vi "triggerModbus.vi"(8 "error in (no error)":errorcluster, 11 "Model in":refnum<class "Model.lvclass">) -> (0 "error out":errorcluster, 3 "Model out":refnum<class "Model.lvclass">)   [LabVIEW 2016, in "Model.lvclass"]
uses:
  Model.lvclass
  Model.lvclass/Model.ctl
  Resources/FPGA/FPGA.lvclass
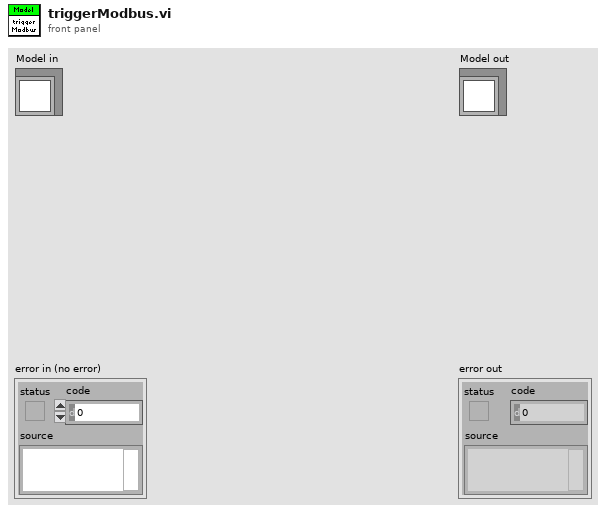
[diagram p1: front panel]
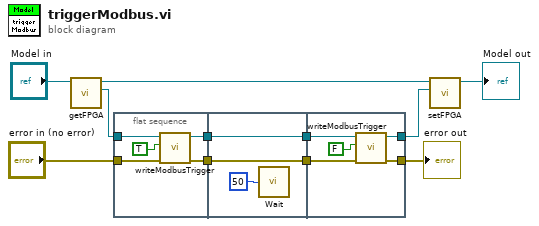
[diagram p0: block diagram]
diagram:
  n1 = call "getFPGA.vi"("Model in"="Model in") -> ("FPGA"=w8:refnum<class "FPGA.lvclass">, "Model out"=w10:refnum<class "Model.lvclass">)  [unwired: 9 in]
  n2 = flat-sequence {
    tunnel: w8 -> [w16]
    tunnel: [w15] -> w6
    tunnel: "error in (no error)" -> [w13]
    tunnel: [w12] -> w2
    tunnel: [w18] -> w7
    tunnel: w6 -> [w18]
    tunnel: [w17] -> w3
    tunnel: w2 -> [w17]
    tunnel: w7 -> [w24]
    tunnel: [w23] -> w5
    tunnel: w3 -> [w21]
    tunnel: [w20] -> w1
    frame #0 {
      n3 = call "writeModbusTrigger.vi"("error in (no error)"=w13, "Trigger"=TRUE, "FPGA in"=w16) -> ("error out"=w12:errorcluster, "FPGA out"=w15:refnum<class "FPGA.lvclass">)  [unwired: 7 in]
    }
    frame #1 {
      n4 = call "Wait"("Count(uSec)"=u32 50) -> ()  [unwired: 1 out]
    }
    frame #2 {
      n5 = call "writeModbusTrigger.vi"("error in (no error)"=w21, "Trigger"=FALSE, "FPGA in"=w24) -> ("error out"=w20:errorcluster, "FPGA out"=w23:refnum<class "FPGA.lvclass">)  [unwired: 7 in]
    }
  }
  n6 = call "setFPGA.vi"("FPGA"=w5, "Model in"=w10) -> ("Model out"=→"Model out":refnum<class "Model.lvclass">)  [unwired: 9 in]
  "error out" <- w1
